vi "NEWTempInterpolate.vi"(9 "method":i32(ring)=3 items=["nearest", "linear", "spline", "cubic Hermite", "Lagrange"], 10 "Ic Arr (Baseline 1st)":dbl[](array[numeric]), 11 "Experimental Temp":dbl[](array[numeric])=[18.4, 18.231891383158448, 18.24049723734947, 18.259872778642375, 18.24327868360467, 18.285287761576594, 18.267463310443883, 18.292538881002926, 18.26554917834413, 18.29602913993646, 18.299730397367085, 18.285885351489057, 18.29062473202634, 18.307624527154363, 18.31540492079139, 18.298020360534316, 18.314668591424958, 18.297115444637694, 18.306811753249328, 18.301513671528042, 18.317842805624867, 18.315006948703175, 18.313207166358232, 18.30859455974554, 18.338016485002793, 18.323649559762128, 18.330676416594006, 18.331785760041782, 18.327341976367798, 18.332722233005153, 18.345021772072965, 18.350327388226887, 18.342169818782516, 18.340500574743867, 18.33843187107747, 18.340878060076584, 18.326166736777683, 18.34697530916811, 18.338558905054587, 18.34718971784488, 18.341070186014875, 18.35805868390169, 18.36893205707957, 18.341370225719213, 18.355426558825627, 18.357781291570642, 18.34492536571592, 18.35393510676855, 18.351103088592172, 18.3534909940848, 18.35682951469931, 18.342291093462634, 18.365377153021686, 18.361111757951804, 18.351891839035062, 18.361527229351477, 18.35940185556197, 18.3615995732063, 18.37372952535344, 18.362301456518782, 18.33656936412912, 18.27623462885558, 18.273574407592296, 18.305337078477002, 18.3126085159451, 18.308089983832204, 18.300238661760176, 18.305583859971488, 18.304462906948054, 18.29534531045821, 18.290148396949274, 18.301496837208486, 18.310746421562868, 18.302543297783323, 18.303864227888997, 18.295833014633857, 18.29568200686066, 18.312866748017914, 18.29000763763878, 18.28821794114912, 18.29682090329953, 18.281245765953763, 18.274812496282376, 18.23288594801176, 18.32231905198581, 18.30964208437325, 18.31498399938971, 18.23226628541555, 18.231654636086216, 18.23615925976504, 18.21345616126718, 18.21837820592867, 18.21860793284998, 18.234277425909983, 18.218773039419013, 18.24416476856648, 18.241676189742396, 18.231824046050487, 18.242226803114498, 18.227380057361508, 18.24592006769532, 18.23192518414921, 18.238726142437162, 18.238244091822768, 18.249526486219004, 18.24178029921277, 18.25669110093001, 18.243753388328738, 18.26323533711218, 18.243448892729887, 18.257224502146336, 18.254303849506492, 18.25215193542844, 18.252640154665748, 18.245545033539976, 18.25879812442158, 18.240834428332697, 18.248242368093784, 18.24406315368215, 18.257909279585473, 18.24833012211465, 18.251543653598304, 18.261777745822865, 18.250122632047425, 18.246481216829608, 18.262359587213535, 18.2539323196966, 18.25763120490675, 18.251991929687865, 18.24178374151219, 18.250400068004648, 18.248393774334794, 18.2374817957138, 18.254033207621486, 18.24317561520175, 18.23482668119551, 18.242655570582155, 18.241155349399737, 18.243598022625026, 18.234191835062457, 18.238824922897972, 18.244390555647772, 18.317274308443736, 18.322441121087905, 18.314355933753063, 18.317390465791632, 18.313132265281922, 18.314177317795032, 18.31835249075461, 18.315749109475387, 18.304481066675496, 18.311324960049603, 18.310140384668628, 18.30411482895721, 18.301385735029964, 18.307949185661883, 18.309664631210723, 18.308931801402498, 18.30949606026504, 18.298667868018114, 18.303109892971552, 18.30680439536865, 18.30087349965061, 18.31424861597566, 18.30255179854429, 18.315788501828653, 18.295102942519545, 18.303266552174538, 18.310060063552044, 18.294777353820212, 18.30221428128795, 18.290934661901645, 18.298308569625576, 18.29266852802786, 18.300864549293888, 18.293246294244234, 18.29678273893539, 18.2915902284584, 18.305428269354437, 18.292676146385414, 18.29431976682345, 18.28851572978196, 18.29387161972831, 18.28045594456895, 18.270365642633067, 18.29167387044146, 18.274684641503875, 18.292261577542384, 18.2887820186869, 18.29023591299448, 18.277952206984708, 18.273093314423424, 18.271572434065774, 18.27608285083385, 18.263613860591253, 18.262530284496364, 18.25273429638152, 18.269741988420975, 18.255724513373156, 18.260636689080414, 18.25078671780851, 18.256525542793053, 18.24150438427882, 18.237337397617264, 18.236146203991552, 18.5, nan]) -> (0 "Temp Data":dbl[](array[numeric]), 1 "Ic Data":dbl[](array[numeric]), 2 "xi used":dbl[](array[numeric]) format="%_6g", 4 "Predicted Temp (C)":dbl[](array[numeric]), 5 "Predicted Temp (K)":dbl[](array[numeric]) format="%_6g")   [LabVIEW 2022 SP3]
uses:
  <vilib>/Utility/file.llb/Read Delimited Spreadsheet (DBL).vi
  <vilib>/gmath/NI_Gmath.lvlib
  <vilib>/Analysis/6fits.llb/Curve Fitting Criteria.ctl
  <vilib>/Analysis/NI_AALPro.lvlib
  <vilib>/Analysis/polynomials.llb/1D Linear Evaluation (DBL).vi
panel:
  out "Loaded Path":path
  out "percentage change 2":dbl[](array[numeric])
  out "Expected Ic Fluct (from baseline) 2":dbl[](array[numeric])
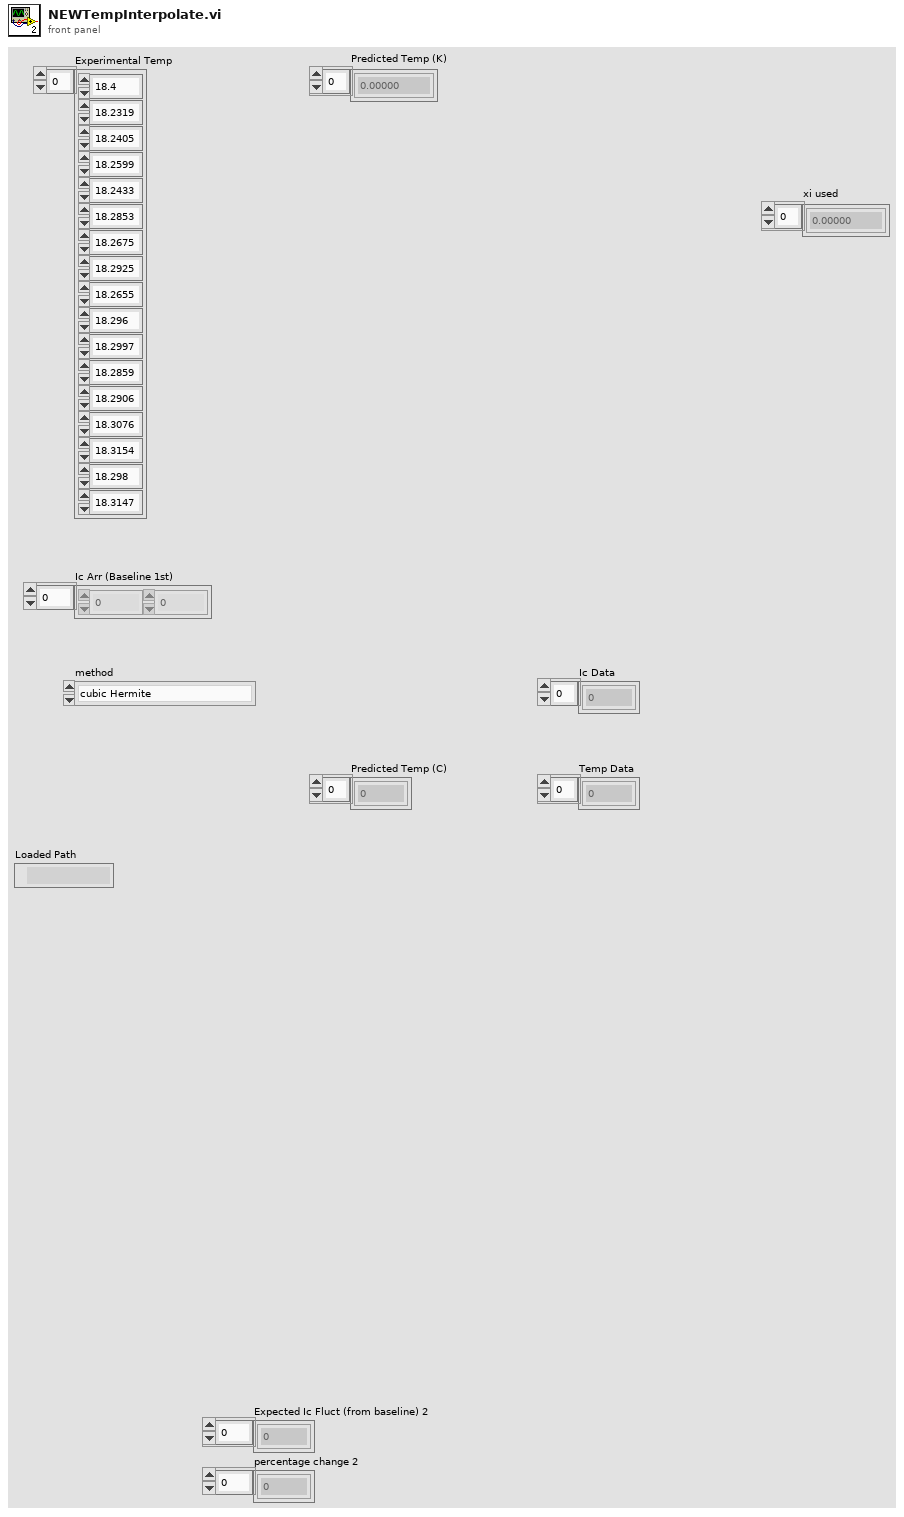
[diagram p1: front panel]
types:
  T1 = typedef "NI_AALPro.lvlib/Curve Fitting Criteria.ctl" = u16
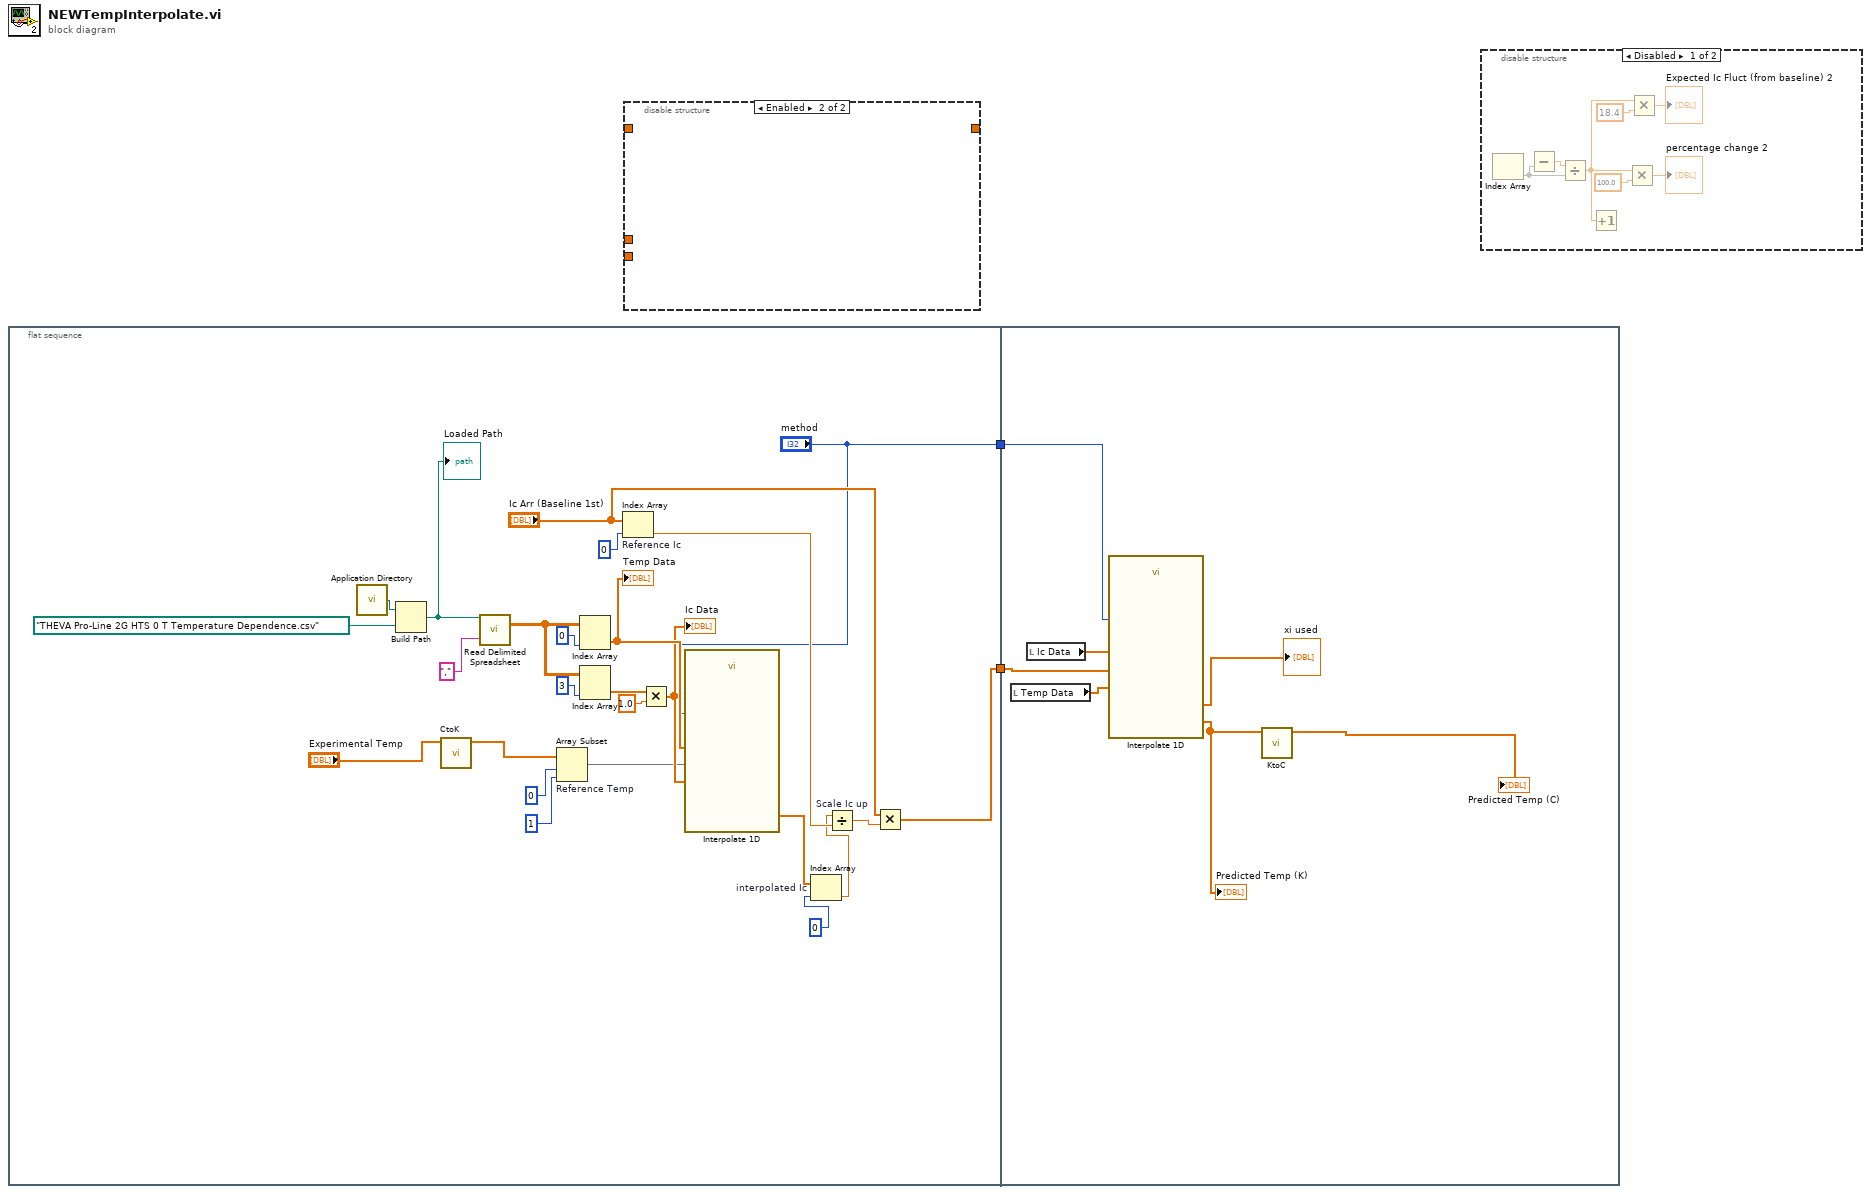
[diagram p0: block diagram]
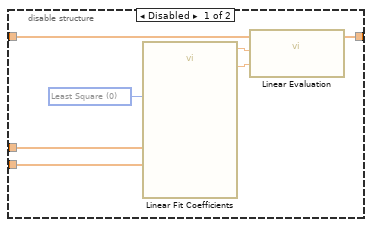
[diagram p2: hidden frame]
diagram:
  n1 = flat-sequence {
    tunnel: [w12] -> w2
    tunnel: ["method"] -> w1
    tunnel: w2 -> [w33]
    tunnel: w1 -> [w31]
    frame #0 {
      n2 = call <vilib>:"Application Directory.vi"() -> ("Application Directory"=w20:path)
      n3 = Build Path(base path=w20, name or relative path=path "THEVA Pro-Line 2G HTS 0 T Temperature Dependence.csv") -> (appended path=w19:path)
      "Loaded Path" <- w19
      n4 = call "CtoK.vi"("C"="Experimental Temp") -> ("K"=w6:dbl[])  [unwired: 10 in]
      n5 = call-poly <vilib>:"Read Delimited Spreadsheet.vi"("file path (dialog if empty)"=w19, "delimiter (\\t)"="," ("delimiter (\\t)")) -> ("all rows"=w27:dbl[][])  [unwired: 8 in, 5 out]
      n6 = Array Subset "Reference Temp"(array=w6, index=0, length=1 ("index")) -> (w9:dbl[])
      n7 = Index Array(array=w27, index (col)=0 ("disabled index (col)")) -> (element=w17:dbl[])  [unwired: 1 in]
      "Temp Data" <- w17
      n8 = Index Array(array=w27, index (col)=3 ("disabled index (col)")) -> (element=w23:dbl[])  [unwired: 1 in]
      n9 = Index Array "Reference Ic"(array="Ic Arr (Baseline 1st)", index=0 ("disabled index (col)")) -> (element=w11:dbl)
      n10 = Multiply(x=w23, y=1.0) -> (x*y=w16:dbl[])
      "Ic Data" <- w16
      n11 = call <vilib>:"Interpolate 1D.vi"("method"="method", "xi"=w9, "X"=w17, "Y"=w16) -> ("yi"=w4:dbl[])  [unwired: 5 in, 2 out]
      n12 = Index Array "interpolated Ic"(array=w4, index=0 ("disabled index (col)")) -> (element=w3:dbl)
      n13 = Divide "Scale Ic up"(x=w3, y=w11) -> (x/y=w10:dbl)
      n14 = Multiply(x="Ic Arr (Baseline 1st)", y=w10) -> (x*y=w12:dbl[])
    }
    frame #1 {
      n15 = local read "Temp Data"() -> (w30:dbl[])
      n16 = local read "Ic Data"() -> (w32:dbl[])
      n17 = call <vilib>:"Interpolate 1D.vi"("method"=w31, "xi"=w33, "X"=w32, "Y"=w30) -> ("xi used"=→"xi used":dbl[], "yi"=w29:dbl[])  [unwired: 5 in, 1 out]
      "Predicted Temp (K)" <- w29
      n18 = call "KtoC.vi"("K"=w29) -> ("C"=→"Predicted Temp (C)":dbl[])  [unwired: 10 in]
    }
  }
  n19 = disable-structure shown="Enabled" {
    disable-tunnel: _ -> [w41 _]
    disable-tunnel: _ -> [w40 _]
    disable-tunnel: _ -> [w37 _]
    disable-tunnel: [w36 _] -> _
    frame Disabled {
      w35 = T1 0 items=["Least Square", "Least Absolute Residual", "Bisquare"] ("method")
      n20 = call <vilib>:"Linear Fit Coefficients.vi"("Y"=w41, "X"=w40, "method"=w35) -> ("slope"=w39:dbl, "intercept"=w38:dbl)  [unwired: 10 in, 1 out]
      n21 = call-poly <vilib>:"Linear Evaluation.vi"("b"=w38, "a"=w39, "X"=w37) -> ("Y[i]=X[i]*a+b"=w36:dbl[])  [unwired: 1 out]
    }
    frame Enabled {
    }
  }
  n22 = disable-structure shown="Disabled" {
    frame Disabled {
      n23 = Index Array() -> (element=w49)  [unwired: 2 in]
      n24 = Subtract(y=w49) -> (x=w48:dbl, x-y=w45:dbl)
      n25 = Divide(x=w45, y=w49) -> (x/y=w43:dbl)
      n26 = Increment(x=w43) -> (x+1=w42:dbl)
      n27 = Multiply(x=w43, y=100.0) -> (x*y=→"percentage change 2":dbl)
      n28 = Multiply(x=w43, y=18.4) -> (x*y=→"Expected Ic Fluct (from baseline) 2":dbl)
    }
    frame Enabled {
    }
  }
